vi "Do.vi"(8 "error in (no error)":errorcluster, 10 "Actor in":refnum<class "Actor.lvclass">, 11 "ppanel_connect_to_hydraharp Msg":refnum<class "ppanel_connect_to_hydraharp Msg.lvclass">) -> (0 "error out":errorcluster, 2 "Actor out":refnum<class "Actor.lvclass">)   [LabVIEW 2015, in "ppanel_connect_to_hydraharp Msg.lvclass"]
doc: "This VI delivers the message to the actor by calling the appropriate method(s) on the actor."
uses:
  ppanel_connect_to_hydraharp Msg.lvclass
  <vilib>/ActorFramework/Actor/Actor.lvclass
  picoharp_panel/picoharp_panel.lvclass
  ppanel_connect_to_hydraharp Msg.lvclass/ppanel_connect_to_hydraharp Msg.ctl
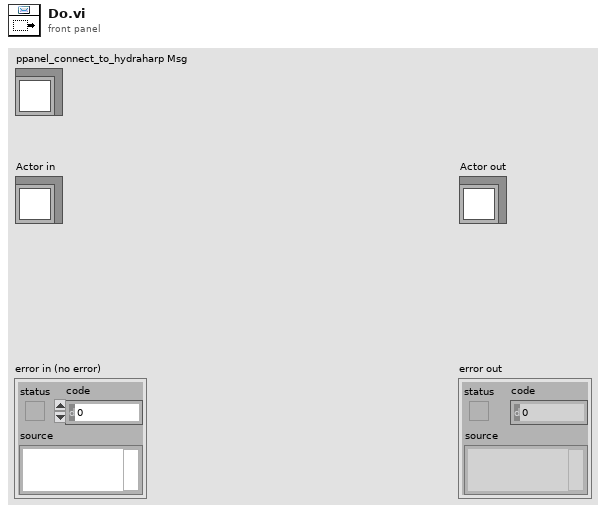
[diagram p1: front panel]
types:
  T1 = typedef "hpanel_hydraharp_settings.ctl" = cluster{"Sync Settings":T2, "CH 1":T4, "CH 2":T4, "CH 3":T4, "CH 4":T4, "binning":i32, "CH 5":T4, "CH 6":T4, "CH 7":T4, "CH 8":T4}
  T2 = typedef "hpanel_sync_settings.ctl" = cluster{"snc_count":i32, "snc_level":i32, "snc_ZeroX":i32, "snc_offs":i32, "sync_div":T3}
  T3 = typedef "hpanel_sync_div.ctl" = enum16{"1", "2", "4", "8"}
  T4 = typedef "hpanel_channel_settings.ctl" = cluster{"ch_counts":i32, "ch_level":i32, "ch_ZeroX":i32, "ch_offs":i32}
  T5 = typedef "hpanel_acq_modes.ctl" = u16
  T6 = typedef "ui_user_events.ctl" = cluster{"update_xy_graph":refnum<user-event>, "update_graph":refnum<user-event>, "update_chart":refnum<user-event>, "update_map":refnum<user-event>, "event_loop_stop":refnum<user-event>, "keep_map":refnum<user-event>}
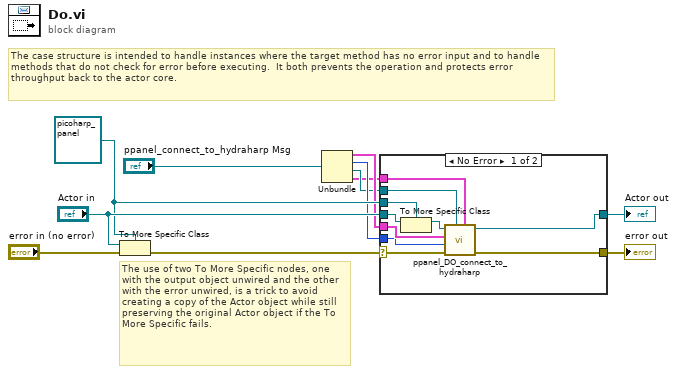
[diagram p0: block diagram]
diagram:
  w5 = refnum<class "picoharp_panel.lvclass"> refnum ("Actor in")
  # "The use of two To More Specific nodes, one with the output object unwired and the other with the error unwired, is a trick to avoid creating a copy of the Actor object while still preserving the original Actor object if the To More Specific fails."
  # "The case structure is intended to handle instances where the target method has no error input and to handle methods that do not check for error before executing.  It both prevents the operation and protects error throughput back to the actor core."
  n1 = To More Specific Class(target class=w5, reference="Actor in", error in="error in (no error)") -> (error out=w9:errorcluster)  [unwired: 1 out]
  n2 = Unbundle("ppanel_connect_to_hydraharp Msg") -> (w4:T1, w3:T5, w2:refnum<user-event>, w1:T6)
  n3 = case shown="No Error" w9 {
    selector: w9 -> [w19 w23]
    tunnel: [w21 w23] -> w8
    tunnel: [w20 w22] -> w7
    tunnel: "Actor in" -> [w18 w22]
    tunnel: w5 -> [w17 _]
    tunnel: w4 -> [w15 _]
    tunnel: w3 -> [w14 _]
    tunnel: w2 -> [w13 _]
    tunnel: w1 -> [w12 _]
    frame No Error {
      n4 = To More Specific Class(target class=w17, reference=w18) -> (specific class reference=w16:refnum<class "picoharp_panel.lvclass">)  [unwired: 1 in, 1 out]
      n5 = call "ppanel_DO_connect_to_hydraharp.vi"("ui_events"=w12, "update_hydraharp_status"=w13, "error in (no error)"=w19, "Mode"=w14, "Hydraharp Settings"=w15, "hydraharp_panel in"=w16) -> ("error out"=w21:errorcluster, "hydraharp_panel out"=w20:refnum<class "picoharp_panel.lvclass">)  [unwired: 4 in]
    }
    frame Error {
      # "If type check fails, pass the original object out again."
    }
  }
  "error out" <- w8
  "Actor out" <- w7
